vi "UIRef.vi"(8 "error in":errorcluster, 11 "HiPOT Channel":refnum<class "HiPOT Channel.lvclass">) -> (0 "error out":errorcluster, 2 "VI refnum":refnum<vi>, 3 "HiPOT Channel out":refnum<class "HiPOT Channel.lvclass">)   [LabVIEW 2025, in "HiPOT.lvlib" / "HiPOT Channel.lvclass"]
doc: "Stores the static reference to the UI of the node.Copyright 2017 National Instruments Corporation\n\nLicensed under the Apache License, Version 2.0 (the \"License\"); you may not use this file except in compliance with the License. You may obtain a copy of the License at http://www.apache.org/licenses/LICENSE-2.0\nUnless required by applicable law or agreed to in writing, software distributed under the License is distributed on an \"AS IS\" BASIS, WITHOUT WARRANTIES OR CONDITIONS OF ANY KIND, either express or implied. See the License for the specific language governing permissions and limitations under the License."
uses:
  HiPOT Channel.lvclass
  HiPOT Channel UI.vi
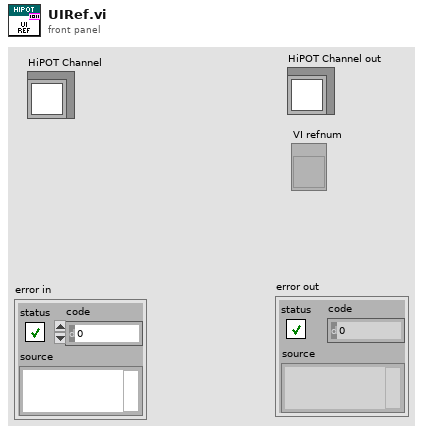
[diagram p1: front panel]
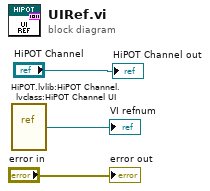
[diagram p0: block diagram]
diagram:
  n1 = vi-ref "HiPOT.lvlib:HiPOT Channel.lvclass:HiPOT Channel UI.vi"() -> (→"VI refnum":refnum<vi>)
  "error out" <- "error in"
  "HiPOT Channel out" <- "HiPOT Channel"
